vi "Uint16 Create.vi"(8 "error in (no error)":errorcluster, 11 "U16 in":u16) -> (0 "error out":errorcluster, 3 "Uint16 DVR out":refnum<data-value>)   [LabVIEW 2010, in "MDSplus.lvlib"]
uses:
  <vilib>/MDSplus/Library/MDSplus.lvlib
  <vilib>/MDSplus/Classes/Data_Class/Scalar_Class/Uint16_Class/Uint16.lvclass
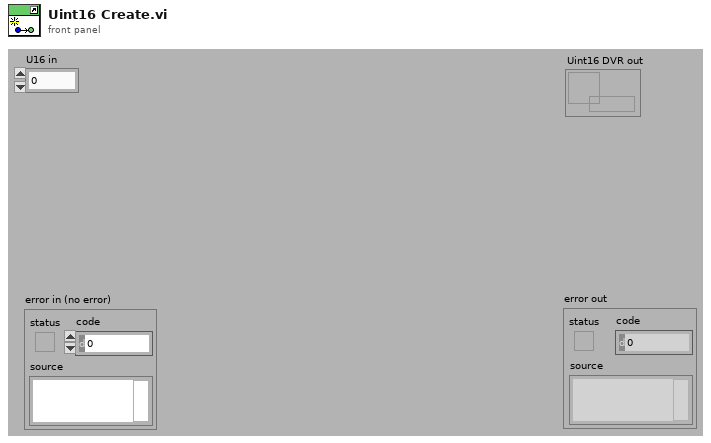
[diagram p1: front panel]
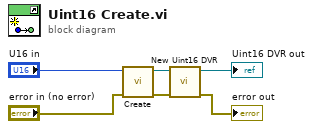
[diagram p0: block diagram]
diagram:
  n1 = call <vilib>:"Create.vi"("error in (no error)"="error in (no error)", "U16 in"="U16 in") -> ("error out"=w3:errorcluster, "Uint16 out"=w4:refnum<class "Uint16.lvclass">)  [unwired: 8 in]
  n2 = call <vilib>:"New Uint16 DVR.vi"("error in (no error)"=w3, "Uint16 in"=w4) -> ("error out"=→"error out":errorcluster, "Uint16 DVR out"=→"Uint16 DVR out":refnum<data-value>)  [unwired: 8 in]
